vi "initiateItems.vi"(8 "error in (no error)":errorcluster, 11 "reference in":refnum<class "Project Panels.lvclass">) -> (0 "error out":errorcluster, 2 "table":T1, 3 "reference out":refnum<class "Project Panels.lvclass">)   [LabVIEW 2015, in "Project Panels.lvclass"]
uses:
  Project Panels.lvclass
  SYS/Items Controller_llb/Items Controller.lvclass
  APP/checkIN_class/checkIN.lvclass
  APP/checkOUT_class/checkOUT.lvclass
  APP/item_class/item.lvclass
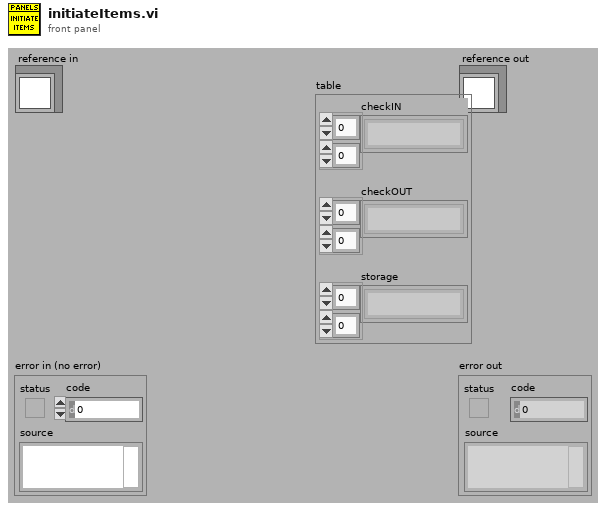
[diagram p1: front panel]
types:
  T1 = cluster{"checkIN":string[][], "checkOUT":string[][], "storage":string[][]}
  T2 = typedef "Project Panels.lvclass/ObjectAttributesRef.ctl" = refnum<data-value>
  T3 = typedef "Project Panels.lvclass/ObjectAttributes.ctl" = cluster{"MyAttribute":dbl, "device_controller_ref":refnum<class "Devices Controller.lvclass">, "file_controller_ref":refnum<class "File Controller.lvclass">, "item_controller_ref":refnum<class "Items Controller.lvclass">, "item_tables":cluster{"checkIN":string[][], "checkOUT":string[][], "storage":string[][]}, "quickbook_table":cluster{"notes":string[][]}, "notification_controller_ref":refnum<class "Notification Controller.lvclass">, "partstracking_controller_ref":refnum<class "PartsTracking Controller.lvclass">, "product_tables":cluster{"k4b2":string[][], "fitmate":string[][], "RMR":string[][], "CPET":string[][], "BP":string[][], "PP":string[][], "k5":string[][], "bb-pft":string[][]}, "rowsColour":u32[], "low_resolution?":bool, "run_python?":bool}
  T4 = cluster{"checkIN_ref":refnum<class "checkIN.lvclass">, "checkOUT_ref":refnum<class "checkOUT.lvclass">, "item_ref":refnum<class "item.lvclass">}
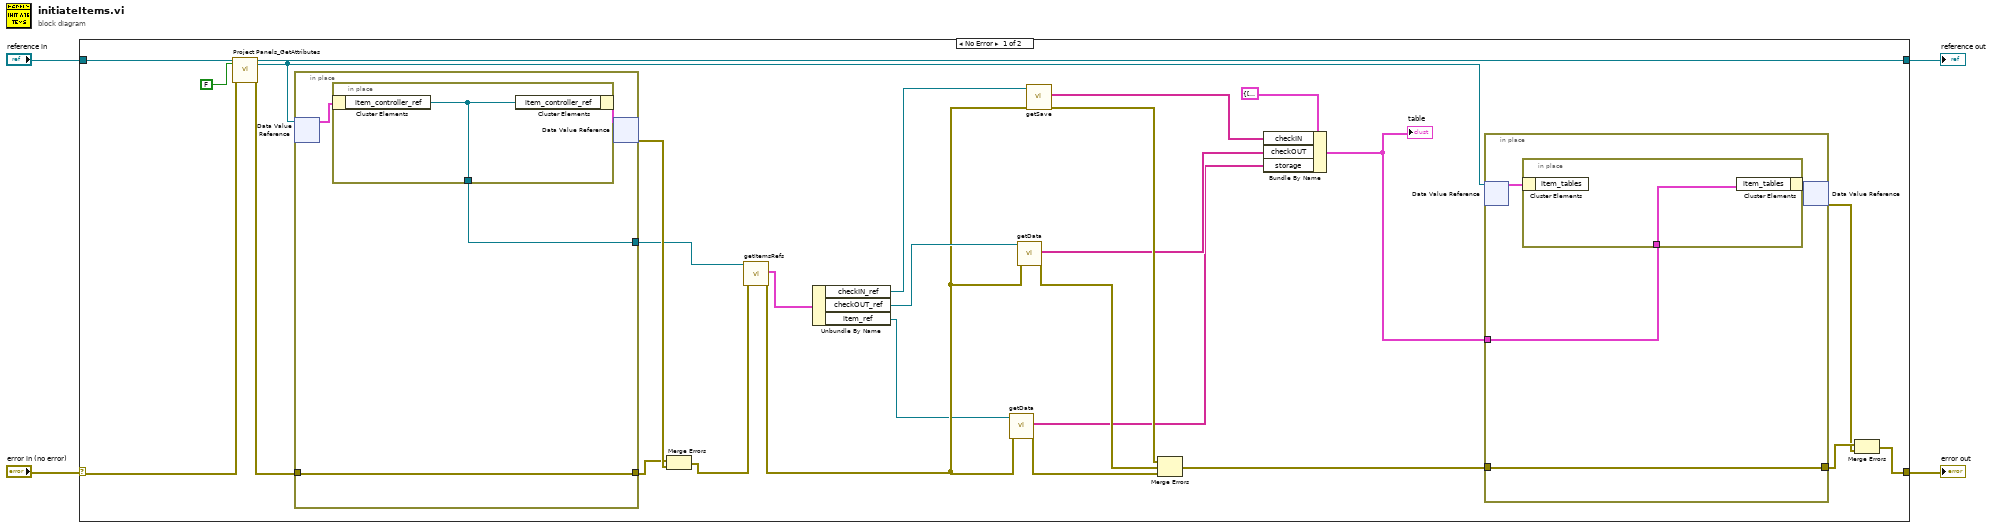
[diagram p0: block diagram]
diagram:
  n1 = case shown="No Error" "error in (no error)" {
    selector: "error in (no error)" -> [w16 w43]
    tunnel: [w18 w43] -> w3
    tunnel: [w26 w42] -> w1
    tunnel: "reference in" -> [w29 w42]
    frame No Error {
      n2 = call "Project Panels_GetAttributes.vi"("reference in"=w29, "return data? (T)"=FALSE, "error in (no error)"=w16) -> ("reference out"=w26:refnum<class "Project Panels.lvclass">, "attributes ref"=w22:T2, "error out"=w27:errorcluster)  [unwired: 13 in, 1 out]
      n3 = in-place {
        in-place-border: w27 -> [w38]
        in-place-border: [w38] -> w30
        in-place-border: [w37] -> w15
        n4 = in-place-dvr #1(w22) -> (w39:T3)  [unwired: 1 out]
        n5 = in-place {
          in-place-border: [w41] -> w37
          n6 = in-place-cluster #2(w39) -> ("item_controller_ref"=w41:refnum<class "Items Controller.lvclass">)
          n7 = in-place-cluster #2("item_controller_ref"=w41) -> (w40:T3)
        }
        n8 = in-place-dvr #1(w40) -> (w31:errorcluster)  [unwired: 1 out]
      }
      n9 = Merge Errors(w30, w31) -> (w24:errorcluster)
      n10 = call "getItemsRefs.vi"("error in (no error)"=w24, "reference in"=w15) -> ("error out"=w8:errorcluster, "itemsRef"=w25:T4)  [unwired: 7 in, 1 out]
      n11 = Unbundle By Name(w25) -> ("checkIN_ref"=w14:refnum<class "checkIN.lvclass">, "checkOUT_ref"=w11:refnum<class "checkOUT.lvclass">, "item_ref"=w6:refnum<class "item.lvclass">)
      n12 = call "getData.vi"("error in (no error)"=w8, "reference in"=w6) -> ("error out"=w7:errorcluster, "data"=w5:string[][])  [unwired: 7 in, 1 out]
      n13 = call "getData.vi"("error in (no error)"=w8, "reference in"=w11) -> ("error out"=w10:errorcluster, "data"=w9:string[][])  [unwired: 7 in, 1 out]
      n14 = call "getSave.vi"("error in (no error)"=w8, "reference in"=w14) -> ("error out"=w12:errorcluster, "data"=w13:string[][])  [unwired: 7 in, 1 out]
      n15 = Merge Errors(w12, w10, w7) -> (w23:errorcluster)
      n16 = Bundle By Name(cluster=T1 {"checkIN"=[], "checkOUT"=[], "storage"=[]} ("item_tables"), "checkIN"=w13, "checkOUT"=w9, "storage"=w5) -> (w21:T1)
      "table" <- w21
      n17 = in-place {
        in-place-border: w23 -> [w33]
        in-place-border: [w33] -> w20
        in-place-border: w21 -> [w32]
        n18 = in-place-dvr #3(w22) -> (w34:T3)  [unwired: 1 out]
        n19 = in-place {
          in-place-border: w32 -> [w36]
          n20 = in-place-cluster #4(w34) -> ()  [unwired: 1 out]
          n21 = in-place-cluster #4("item_tables"=w36) -> (w35:T3)
        }
        n22 = in-place-dvr #3(w35) -> (w19:errorcluster)  [unwired: 1 out]
      }
      n23 = Merge Errors(w20, w19) -> (w18:errorcluster)
    }
    frame Error {
    }
  }
  "error out" <- w3
  "reference out" <- w1
